vi "Save to TDMS.vi"(4 "Stop Time":dbl[unit]=0.1, 6 "Start Time":dbl[unit]=-0.1, 8 "Error In":errorcluster, 9 "Quench Channel":i32, 10 "Quench Start":dbl[unit], 11 "KIT-QA in":refnum<class "KIT-QA.lvclass">) -> (0 "Error Out":errorcluster, 3 "KIT-QA out":refnum<class "KIT-QA.lvclass">)   [LabVIEW 2015, in "KIT-QA.lvlib" / "KIT-QA.lvclass"]
doc: "Save quench data to TDMS."
uses:
  KIT-QA.lvclass
  KIT-QA.lvclass/KIT-QA.ctl
  <vilib>/Waveform/WDTOps.llb/WDT Get XY Value DBL.vi
  <vilib>/Waveform/WDTOps.llb/WDT Waveform Duration DBL.vi
  <vilib>/Waveform/WDTOps.llb/WDT Get Waveform Subset DBL.vi
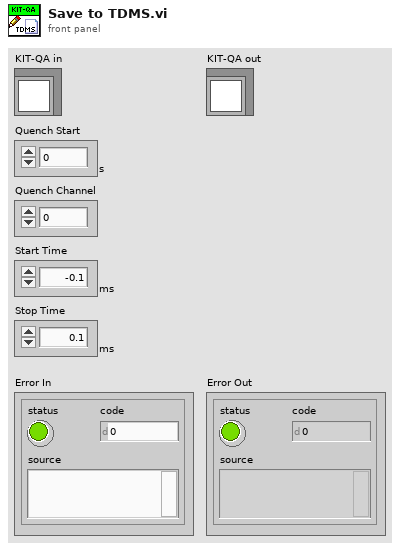
[diagram p1: front panel]
types:
  T1 = enum16{"open", "open or create", "create or replace", "create", "open (read-only)"}
  T2 = cluster{"timestamps":timestamp[], "data":dbl[]}[]
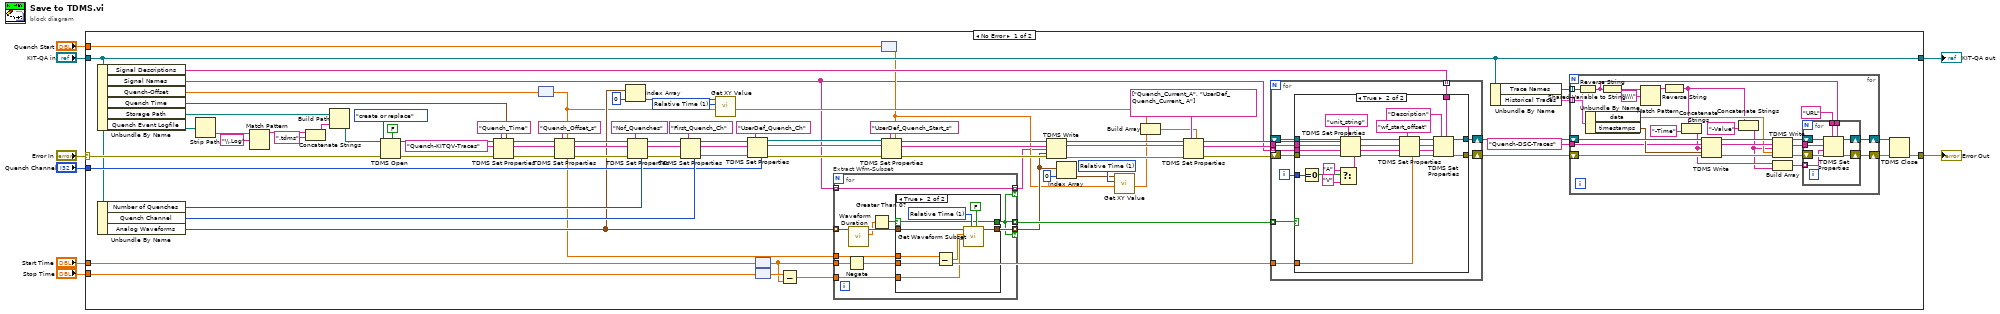
[diagram p0: block diagram]
diagram:
  n1 = case shown="No Error" "Error In" {
    selector: "Error In" -> [w79 w184]
    tunnel: [w78 w184] -> w7
    tunnel: [w37 w183] -> w5
    tunnel: "KIT-QA in" -> [w37 w183]
    tunnel: "Quench Start" -> [w73 _]
    tunnel: "Quench Channel" -> [w52 _]
    tunnel: "Start Time" -> [w51 _]
    tunnel: "Stop Time" -> [w50 _]
    frame No Error {
      w16 = u16 1 items=["Samples", "Relative Time"] ("Y position format")
      w21 = u16 1 items=["Samples", "Relative Time"] ("Y position format")
      n2 = Unbundle By Name(w37) -> ("Signal Descriptions"=w60:string[], "Signal Names"=w10:string[], "Quench-Offset"=w61:dbl[unit], "Quench Time"=w67:timestamp, "Storage Path"=w75:path, "Quench Event Logfile"=w80:path)
      n3 = Unbundle By Name(w37) -> ("Number of Quenches"=w77:i32, "Quench Channel"=w76:i32, "Analog Waveforms"=w20:waveform(dbl)[])
      n4 = Strip Path(path=w80) -> (name=w90:string)  [unwired: 1 out]
      n5 = Match Pattern(string=w90, regular expression="\\.Log") -> (before substring=w88:string)  [unwired: 1 in, 3 out]
      n6 = Concatenate Strings(w88, ".tdms" ("string")) -> (w86:string)
      n7 = Build Path(base path=w75, name or relative path=w86) -> (appended path=w85:path)
      n8 = TDMS Open(5:FALSE ("create index file? (T)"), 8:w79, 10:T1."create or replace" ("operation (0:open)"), 11:w85) -> (0:w68:errorcluster, 3:w69:refnum<k34>)  [unwired: 3 in]
      n9 = TDMS Set Properties(5:w67, 7:"Quench_Time", 8:w68, 10:"Quench-KITQV-Traces" ("group name"), 11:w69) -> (0:w64:errorcluster, 2:w43:string, 3:w65:refnum<k34>)  [unwired: 1 in, 1 out]
      n10 = node(w61) -> (w19:dbl)
      n11 = TDMS Set Properties(5:w19, 7:"Quench_Offset_s", 8:w64, 10:w43, 11:w65) -> (0:w62:errorcluster, 2:w42:string, 3:w63:refnum<k34>)  [unwired: 1 in, 1 out]
      n12 = Index Array(array=w20, index=0) -> (element=w22:waveform(dbl))
      n13 = TDMS Set Properties(5:w77, 7:"Nof_Quenches", 8:w62, 10:w42, 11:w63) -> (0:w71:errorcluster, 2:w41:string, 3:w72:refnum<k34>)  [unwired: 1 in, 1 out]
      n14 = TDMS Set Properties(5:w76, 7:"First_Quench_Ch", 8:w71, 10:w41, 11:w72) -> (0:w53:errorcluster, 2:w40:string, 3:w54:refnum<k34>)  [unwired: 1 in, 1 out]
      n15 = call-poly <vilib>:"Get XY Value.vi"("Y position"=w19, "Y position format"=w21, "waveform in"=w22) -> ("Y value"=w18:dbl)  [unwired: 4 in, 4 out]
      n16 = TDMS Set Properties(5:w52, 7:"UserDef_Quench_Ch", 8:w53, 10:w40, 11:w54) -> (0:w45:errorcluster, 2:w39:string, 3:w46:refnum<k34>)  [unwired: 1 in, 1 out]
      n17 = node(w51) -> (w48:dbl)
      n18 = node(w50) -> (w49:dbl)
      n19 = Subtract(x=w49, y=w48) -> (x-y=w47:dbl)
      n20 = for "Extract Wfm-Subset" {
        tunnel: w20 -> [w169] mode=indexing
        tunnel: w19 -> [w170]
        tunnel: [w171] -> w13 mode=indexing if=w161
        tunnel: w48 -> [w165]
        tunnel: [w161] -> w56 mode=indexing
        tunnel: w47 -> [w163]
        tunnel: w10 -> [w162] mode=indexing
        tunnel: [w162] -> w9 mode=indexing if=w161
        n21 = Negate(x=w165) -> (-x=w164:dbl)
        n22 = call-poly <vilib>:"Waveform Duration.vi"("waveform in"=w169) -> ("duration"=w167:dbl, "waveform out"=w168:waveform(dbl))  [unwired: 8 in, 1 out]
        n23 = Greater Than 0?(x=w167) -> (x > 0?=w166:bool)
        n24 = case shown="True" w166 {
          selector: w166 -> [w172 w176]
          tunnel: [w173 w179] -> w171
          tunnel: w170 -> [_ w178]
          tunnel: w168 -> [w173 w177]
          tunnel: [w172 w176] -> w161
          tunnel: w164 -> [_ w175]
          tunnel: w163 -> [_ w174]
          frame False {
          }
          frame True {
            w181 = u16 1 items=["Samples", "Relative Time"] ("start/duration format")
            n25 = Subtract(x=w178, y=w175) -> (x-y=w182:dbl)
            n26 = call-poly <vilib>:"Get Waveform Subset.vi"("open interval? (T)"=FALSE, "start/duration format"=w181, "duration"=w174, "start samples/time"=w182, "waveform in"=w177) -> ("waveform out"=w179:waveform(dbl))  [unwired: 1 in, 3 out]
          }
        }
      }
      n27 = node(w73) -> (w12:dbl)
      n28 = TDMS Set Properties(5:w12, 7:"UserDef_Quench_Start_s", 8:w45, 10:w39, 11:w46) -> (0:w58:errorcluster, 2:w38:string, 3:w59:refnum<k34>)  [unwired: 1 in, 1 out]
      n29 = TDMS Write(0:w59, 5:w38, 7:w9, 9:w13, 11:w58) -> (4:w57:refnum<k34>, 6:w28:string, 15:w29:errorcluster)  [unwired: 1 in, 1 out]
      n30 = Index Array(array=w13, index=0) -> (element=w15:waveform(dbl))
      n31 = call-poly <vilib>:"Get XY Value.vi"("Y position"=w12, "Y position format"=w16, "waveform in"=w15) -> ("Y value"=w11:dbl)  [unwired: 4 in, 4 out]
      n32 = Build Array(w18, w11) -> (w17:dbl[])
      n33 = TDMS Set Properties(5:w17, 7:string[] ["Quench_Current_A", "UserDef_Quench_Current_ A"] ("property names"), 8:w29, 10:w28, 11:w57) -> (0:w24:errorcluster, 2:w23:string, 3:w25:refnum<k34>)  [unwired: 1 in, 1 out]
      n34 = for {
        tunnel: w10 -> [w128] mode=indexing
        shift-right: [w127] -> w36
        shift-left: w25 -> [w131]
        shift-right: [w126] -> w35
        shift-left: w24 -> [w130]
        tunnel: w23 -> [w129]
        tunnel: w60 -> [w134] mode=indexing
        tunnel: w48 -> [w132]
        tunnel: w56 -> [w125] mode=indexing
        i -> [w133]
        n35 = case shown="True" w125 {
          tunnel: w134 -> [_ w160]
          tunnel: w133 -> [_ w159]
          tunnel: w132 -> [_ w150]
          tunnel: w131 -> [w136 w146]
          tunnel: w130 -> [w135 w145]
          tunnel: w129 -> [_ w144]
          tunnel: w128 -> [_ w143]
          tunnel: [w136 w138] -> w127
          tunnel: [w135 w137] -> w126
          frame False {
          }
          frame True {
            n36 = Equal To 0?(x=w159) -> (x = 0?=w158:bool)
            n37 = Select(t="A", s=w158, f="V") -> (s? t:f=w155:string)
            n38 = TDMS Set Properties(5:w155, 7:"unit_string", 8:w145, 9:w143, 10:w144, 11:w146) -> (0:w139:errorcluster, 1:w140:string, 2:w141:string, 3:w142:refnum<k34>)
            n39 = TDMS Set Properties(5:w150, 7:"wf_start_offset", 8:w139, 9:w140, 10:w141, 11:w142) -> (0:w152:errorcluster, 1:w153:string, 2:w154:string, 3:w151:refnum<k34>)
            n40 = TDMS Set Properties(5:w160, 7:"Description", 8:w152, 9:w153, 10:w154, 11:w151) -> (0:w137:errorcluster, 3:w138:refnum<k34>)  [unwired: 2 out]
          }
        }
      }
      n41 = Unbundle By Name(w37) -> ("Trace Names"=w32:refnum<k21>[], "Historical Traces"=w30:T2)
      n42 = for {
        tunnel: "Quench-DSC-Traces" ("group name") -> [w103]
        tunnel: w32 -> [w97] mode=indexing
        tunnel: w30 -> [w113] mode=indexing
        shift-right: [w100] -> w34
        shift-left: w36 -> [w116]
        shift-right: [w98] -> w31
        shift-left: w35 -> [w115]
        n43 = Shared Variable to String(1:w97) -> (0:w95:string)
        n44 = Unbundle By Name(w113) -> ("data"=w105:dbl[], "timestamps"=w106:timestamp[])
        n45 = Reverse String(1:w95) -> (0:w110:string)
        n46 = Match Pattern(string=w110, regular expression="\\\\") -> (before substring=w109:string)  [unwired: 1 in, 3 out]
        n47 = Reverse String(1:w109) -> (0:w101:string)
        n48 = Concatenate Strings(w101, "-Time" ("string")) -> (w93:string)
        n49 = TDMS Write(0:w116, 5:w103, 7:w93, 9:w106, 11:w115) -> (4:w112:refnum<k34>, 6:w107:string, 15:w111:errorcluster)  [unwired: 1 in, 1 out]
        n50 = Concatenate Strings(w101, "-Value" ("string")) -> (w92:string)
        n51 = TDMS Write(0:w112, 5:w107, 7:w92, 9:w105, 11:w111) -> (4:w114:refnum<k34>, 6:w94:string, 15:w99:errorcluster)  [unwired: 1 in, 1 out]
        n52 = Build Array(w93, w92) -> (w91:string[])
        n53 = for {
          tunnel: "URL" ("string") -> [w120]
          tunnel: w95 -> [w119]
          tunnel: w94 -> [w118]
          shift-right: [w123] -> w100
          shift-left: w114 -> [w124]
          shift-right: [w121] -> w98
          shift-left: w99 -> [w122]
          tunnel: w91 -> [w117] mode=indexing
          n54 = TDMS Set Properties(5:w119, 7:w120, 8:w122, 9:w117, 10:w118, 11:w124) -> (0:w121:errorcluster, 3:w123:refnum<k34>)  [unwired: 2 out]
        }
      }
      n55 = TDMS Close(8:w31, 11:w34) -> (0:w78:errorcluster)  [unwired: 1 out]
    }
    frame Error {
    }
  }
  "Error Out" <- w7
  "KIT-QA out" <- w5
